vi "tm_getframe16_40.vi"(6 "View":i32(ring) items=["default"=0, "view 1"=1048576, "view 2"=2097152, "view 3"=3145728, "view 4"=4194304], 7 "Options":i32(ring) items=["no option"=0, "high contrast"=16], 8 "error in (no error)":errorcluster {"code" format="%.0x"}, 10 "Frame Index":i32=-1, 11 "Handle in":u32) -> (0 "error out":errorcluster {"code" format="%.0x"}, 1 "Timestamp":dbl, 2 "Data":u16[][](array[numeric]), 3 "Handle out":u32)   [LabVIEW 2023]
uses:
  tmcamcon.dll
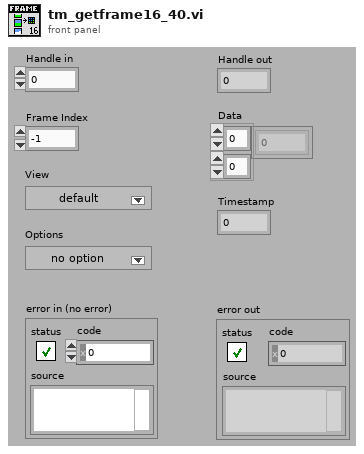
[diagram p1: front panel]
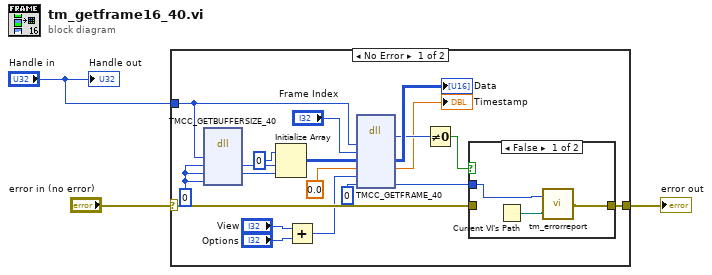
[diagram p0: block diagram]
diagram:
  n1 = case shown="No Error" "error in (no error)" {
    selector: "error in (no error)" -> [w20 w27]
    tunnel: [w19 w27] -> w2
    tunnel: "Handle in" -> [w8 _]
    frame No Error {
      w7 = 0
      n2 = dll-call lib="tmcamcon.dll" fn="TMCC_GETBUFFERSIZE_40"("index"=w8, "height"=w7, "width"=w7, "Erval"=w7) -> ("height"=w10:i32, "width"=w9:i32)  [unwired: 6 in, 2 out]
      n3 = Initialize Array(u16 0, w10, w9) -> (w14:u16[][])
      n4 = Add(x="View", y="Options") -> (x+y=w4:i32)
      n5 = dll-call lib="tmcamcon.dll" fn="TMCC_GETFRAME_40"("index"=w8, "frameindex"="Frame Index", "imgarray"=w14, "timestamp"=0.0, "option"=w4, "Erval"=0) -> ("return type"=w13:u32, "imgarray"=→"Data":u16[][], "timestamp"=→"Timestamp":dbl, "Erval"=w18:i32)  [unwired: 6 in, 2 out]
      n6 = Not Equal To 0?(x=w13) -> (x != 0?=w17:bool)
      n7 = case shown="False" w17 {
        tunnel: w20 -> [_ w26]
        tunnel: [w23 w26] -> w19
        tunnel: w18 -> [w24 _]
        frame False {
          n8 = Current VI's Path() -> (path=w25:path)
          n9 = call "tm_errorreport.vi"("Source"=w25, "Error"=w24) -> ("error out"=w23:errorcluster)
        }
        frame True {
        }
      }
    }
    frame Error {
    }
  }
  "error out" <- w2
  "Handle out" <- "Handle in"
